vi "Test_Spectrum_Name_With_Accums.vi"(8 "Acquis Number":i32, 9 "Accum Number":i32, 10 "Next Spectrum Number":string, 11 "Path of the Day":path) -> (3 "chemin complet":path)   [LabVIEW 2018]
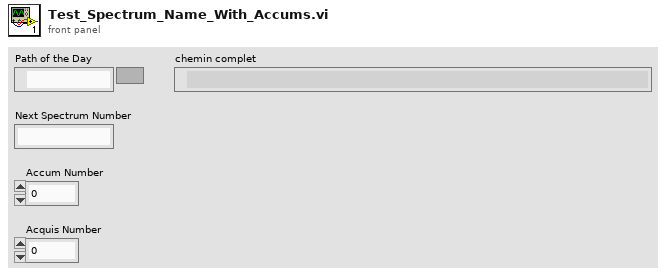
[diagram p1: front panel]
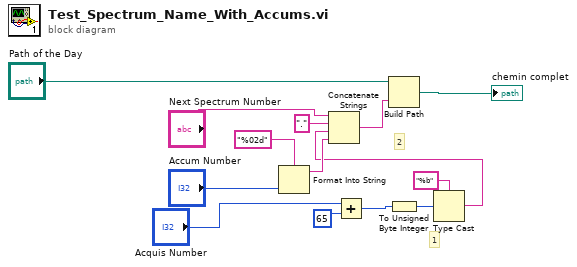
[diagram p0: block diagram]
diagram:
  # "2"
  # "1"
  n1 = Format Into String(format string="%02d" ("chaîne de format"), "Accum Number") -> (resulting string=w8:string)  [unwired: 2 in, 1 out]
  n2 = Add(x="Acquis Number", y=i16 65) -> (x+y=w4:i32)
  n3 = To Unsigned Byte Integer(number=w4) -> (unsigned 8bit integer=w3:u8)
  n4 = Type Cast(type="%b", x=w3) -> (*(type *) &x=w6:string)
  n5 = Concatenate Strings("Next Spectrum Number", "." ("chaîne"), w6, w8) -> (w9:string)
  n6 = Build Path(base path="Path of the Day", name or relative path=w9) -> (appended path=→"chemin complet":path)
